vi "PassFailUUT (SubVI).vi"(8 "error in (no error)":errorcluster, 11 "Table in":refnum<vi>) -> (0 "error out":errorcluster, 3 "PassFaileUUTresult":bool)   [LabVIEW 2017]
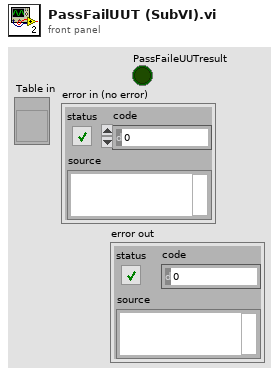
[diagram p1: front panel]
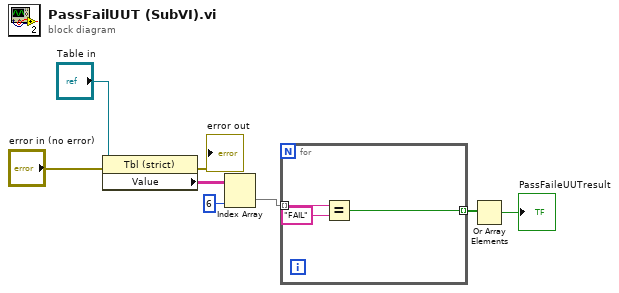
[diagram p0: block diagram]
diagram:
  n1 = property class="Tbl (strict)"(reference="Table in", error in="error in (no error)") -> (error out=→"error out":errorcluster, "Value"=w7:string[][])  [unwired: 1 out]
  n2 = Index Array(array=w7, index (col)=6 ("disabled index (col)")) -> (element=w5:string[])  [unwired: 1 in]
  n3 = for {
    tunnel: w5 -> [w11] mode=indexing
    tunnel: [w9] -> w4 mode=indexing
    n4 = Equal?(x=w11, y="FAIL") -> (x = y?=w9:bool)
  }
  n5 = Or Array Elements(Boolean array=w4) -> (logical OR=→"PassFaileUUTresult":bool)
